vi "machine vision shell VI - initial detection.vi"() -> ()   [LabVIEW 2014]
uses:
  <vilib>/vision/Image Controls.llb/IMAQ Image.ctl
panel:
  in  "Reduced ROI":dbl[](array[numeric])
  in  "Arc limits":dbl[](array[numeric])
  out "obscuration in treatment area":bool
  out "tracking error":bool
  out "detection error":bool
  in  "Corneal rim parameters":dbl[](array[numeric])
  in  "Obscuration ROI size [pixels]":dbl
  in  "Treatment location [pixels]":dbl
  in  "Image ROI":dbl[](array[numeric])
  in  "Image":T1
  # "Inputs"
  # "Outputs"
  # "Center x\n\nCenter y\n\nradios x\n\nradius y"
  # "top left pixel x\n\ntop left pixel y\n\nsize x\n\nsize y"
  # "Left limit angle\n\nRight limit angle"
  # "top left pixel x\n\ntop left pixel y\n\nsize x\n\nsize y"
  # "If binning or any other algorithmic method is used for optimization or reliability, it would be best to add them here.\nAlso, if there are variables that might be used for debugging, adding them here as optionals would be a good idea"
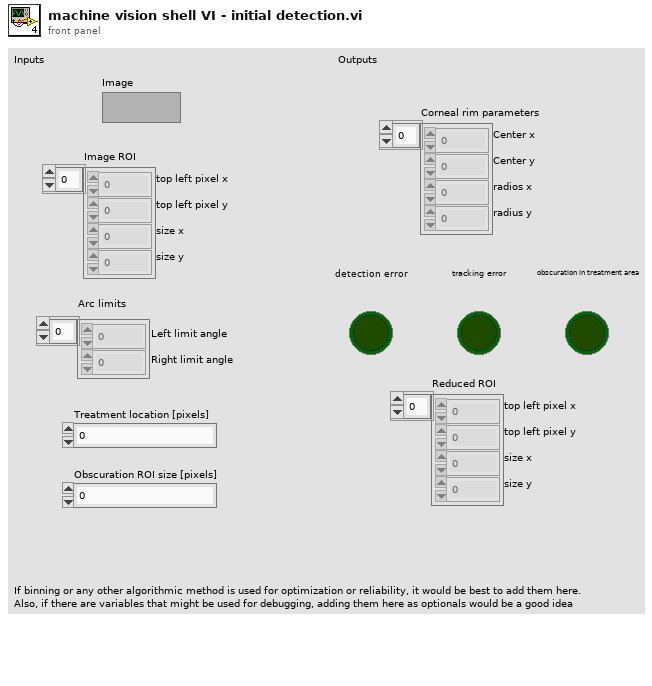
[diagram p1: front panel]
types:
  T1 = typedef "IMAQ Image.ctl" = refnum<image>
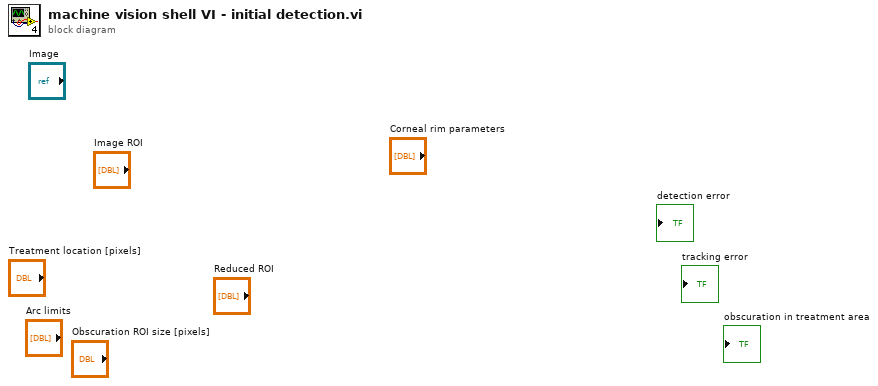
[diagram p0: block diagram]
diagram:
